vi "Get Class.vi"(8 "error in (no error)":errorcluster, 10 "default":refnum<class "Base Interface.lvclass">, 11 "PV Data in":refnum<class "PV Data.lvclass">) -> (0 "error out":errorcluster, 2 "Value out":refnum<class "Base Interface.lvclass">, 3 "PV Data out":refnum<class "PV Data.lvclass">)   [LabVIEW 2020, in "PV Access.lvlib" / "PV Data.lvlib" / "PV Data.lvclass"]
uses:
  PV Data.lvclass
  NT Scalar/NT Scalar.lvclass
  NT Scalar (Numeric)/NT Scalar (Numeric).lvclass
  NT Enum/NT Enum.lvclass
  PV Data.lvclass/PV Data.ctl
  C:/Users/eyw68381/source/repos/pvaccess-labview/labview/source/PV Data/NT Base/NT Base.lvclass
  C:/Users/eyw68381/source/repos/pvaccess-labview/labview/source/PV Data/Base/Base.lvclass
  C:/Users/eyw68381/source/repos/pvaccess-labview/labview/source/PV Data/Base Interface/Base Interface.lvclass
  C:/Users/eyw68381/source/repos/pvaccess-labview/labview/source/PV Data/Has Alarm/Has Alarm.lvclass
  C:/Users/eyw68381/source/repos/pvaccess-labview/labview/source/PV Data/Has Time Stamp/Has Time Stamp.lvclass
  C:/Users/eyw68381/source/repos/pvaccess-labview/labview/source/PV Data/NT Scalar/NT Scalar.lvclass
  C:/Users/eyw68381/source/repos/pvaccess-labview/labview/source/PV Data/Has Alarm Limits/Has Alarm Limits.lvclass
  C:/Users/eyw68381/source/repos/pvaccess-labview/labview/source/PV Data/Has Control Limits/Has Control Limits.lvclass
  C:/Users/eyw68381/source/repos/pvaccess-labview/labview/source/PV Data/NT Scalar (Numeric)/NT Scalar (Numeric).lvclass
  C:/Users/eyw68381/source/repos/pvaccess-labview/labview/source/PV Data/NT Enum/NT Enum.lvclass
  Base Interface/Base Interface.lvclass
  PV Data.lvlib
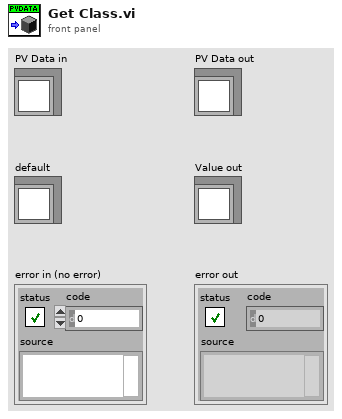
[diagram p1: front panel]
types:
  T1 = typedef "PV Access.lvlib/PV Data.lvlib/Type Code.ctl" = enum8{"Null", "Bool", "BoolA", "Int8", "Int8A", "Int16", "Int16A", "Int32", "Int32A", "Int64", "Int64A", "UInt8", "UInt8A", "UInt16", "UInt16A", "UInt32", "UInt32A", "UInt64", "UInt64A", "Float32", "Float32A", "Float64", "Float64A", "String", "StringA", "Struct", "StructA", "Union", "UnionA", "Any", "AnyA"}
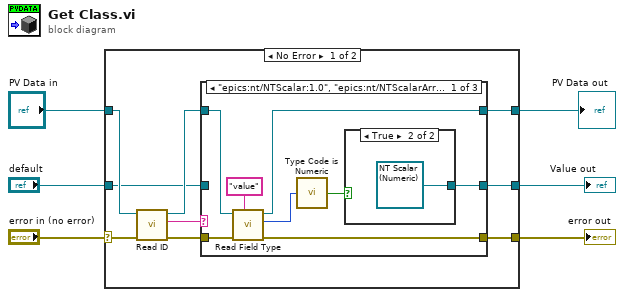
[diagram p0: block diagram]
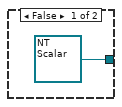
[diagram p2: hidden frame]
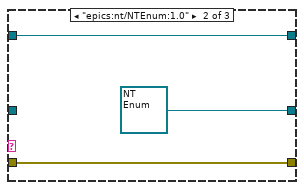
[diagram p3: hidden frame]
diagram:
  n1 = case shown="No Error" "error in (no error)" {
    selector: "error in (no error)" -> [w15 w34]
    tunnel: [w9 w34] -> w2
    tunnel: "PV Data in" -> [w14 w33]
    tunnel: [w10 w33] -> w5
    tunnel: [w8 w32] -> w4
    tunnel: "default" -> [w7 w32]
    frame No Error {
      n2 = call "Read ID.vi"("error in (no error)"=w15, "PV Data in"=w14) -> ("error out"=w11:errorcluster, "ID"=w13:string, "PV Data out"=w12:refnum<class "PV Data.lvclass">)  [unwired: 7 in]
      n3 = case shown="\"epics:nt/NTScalar:1.0\", \"epics:nt/NTScalarArray:1.0\"" w13 {
        tunnel: w12 -> [w22 w28 w31]
        tunnel: [w16 w26 w30] -> w9
        tunnel: w11 -> [w23 w26 w30]
        tunnel: [w18 refnum<class "NT Enum.lvclass"> refnum ("Value.lvlib:NT Scalar (Numeric).lvclass") w29] -> w8
        tunnel: [w17 w28 w31] -> w10
        tunnel: w7 -> [_ _ w29]
        frame "epics:nt/NTScalar:1.0", "epics:nt/NTScalarArray:1.0" {
          n4 = call "Read Field Type.vi"("field name"="value", "error in (no error)"=w23, "PV Data in"=w22) -> ("error out"=w16:errorcluster, "type code"=w20:T1, "PV Data out"=w17:refnum<class "PV Data.lvclass">)  [unwired: 6 in]
          n5 = call "Type Code is Numeric.vi"("type code"=w20) -> ("is match?"=w19:bool)
          n6 = case shown="True" w19 {
            tunnel: [refnum<class "NT Scalar.lvclass"> refnum ("Value.lvlib:NT Scalar.lvclass") refnum<class "NT Scalar (Numeric).lvclass"> refnum ("Value.lvlib:NT Scalar (Numeric).lvclass")] -> w18
            frame False {
            }
            frame True {
            }
          }
        }
        frame "epics:nt/NTEnum:1.0" {
        }
        frame Default {
        }
      }
    }
    frame Error {
    }
  }
  "error out" <- w2
  "PV Data out" <- w5
  "Value out" <- w4
